vi "svx_Polar_Draw_Scale_Line.vi"(8 "grid measurements":T1 {"end angle" format="%.2f"; "start angle" format="%.2f"; "scale factors"."b" format="%.2f"; "scale factors"."a" format="%.2f"}, 10 "decade specs":cluster{"radius":i16, "label":string}[](array[cluster]), 11 "picture":picture) -> (3 "new picture":picture)   [LabVIEW 2017, in "SVX Polar Plot.xctl"]
uses:
  <vilib>/addons/_XControls/Polar Plot/SVX Polar Plot.xctl
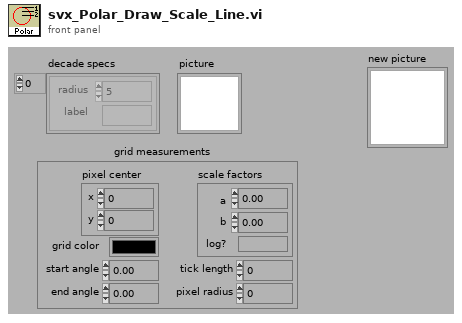
[diagram p1: front panel]
types:
  T1 = cluster{"pixel center":cluster{"x":i16, "y":i16}, "scale factors":cluster{"a":dbl, "b":dbl, "log?":bool}, "grid color":u32, "start angle":dbl, "end angle":dbl, "tick length":i16, "pixel radius":i32}
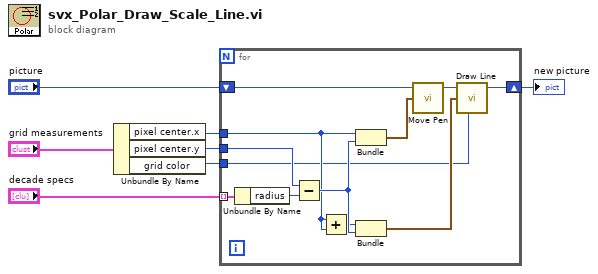
[diagram p0: block diagram]
diagram:
  n1 = Unbundle By Name("grid measurements") -> ("pixel center.x"=w4:i16, "pixel center.y"=w3:i16, "grid color"=w1:u32)
  n2 = for {
    tunnel: "decade specs" -> [w19] mode=indexing
    shift-right: [w16] -> w2
    shift-left: "picture" -> [w18]
    tunnel: w4 -> [w9]
    tunnel: w3 -> [w15]
    tunnel: w1 -> [w8]
    n3 = Unbundle By Name(w19) -> ("radius"=w14:i16)
    n4 = Subtract(x=w15, y=w14) -> (x-y=w13:i16)
    n5 = Add(x=w9, y=w9) -> (x+y=w12:i16)
    n6 = Bundle("x"=w9, w13) -> (w10:cluster{"x":i16, i16})  [unwired: 1 in]
    n7 = Bundle(w12, w13) -> (w11:cluster{i16, i16})  [unwired: 1 in]
    n8 = call <vilib>:"Move Pen.vi"("new position"=w10, "picture"=w18) -> ("new picture"=w17:picture)  [unwired: 3 in]
    n9 = call <vilib>:"Draw Line.vi"("picture"=w17, "end point"=w11, "color(black)"=w8) -> ("new picture"=w16:picture)  [unwired: 6 in]
  }
  "new picture" <- w2
